vi "json editor worksheet.vi"() -> ()   [LabVIEW 2020]
uses:
  controls/step.ctl
  controls/step_type.ctl
  controls/write_read.ctl
panel:
  in  "exit without saving":bool
  in  "steps array out":T1[](array[typedef]) {"value" format="%.2f"}
  in  "exit and save":bool
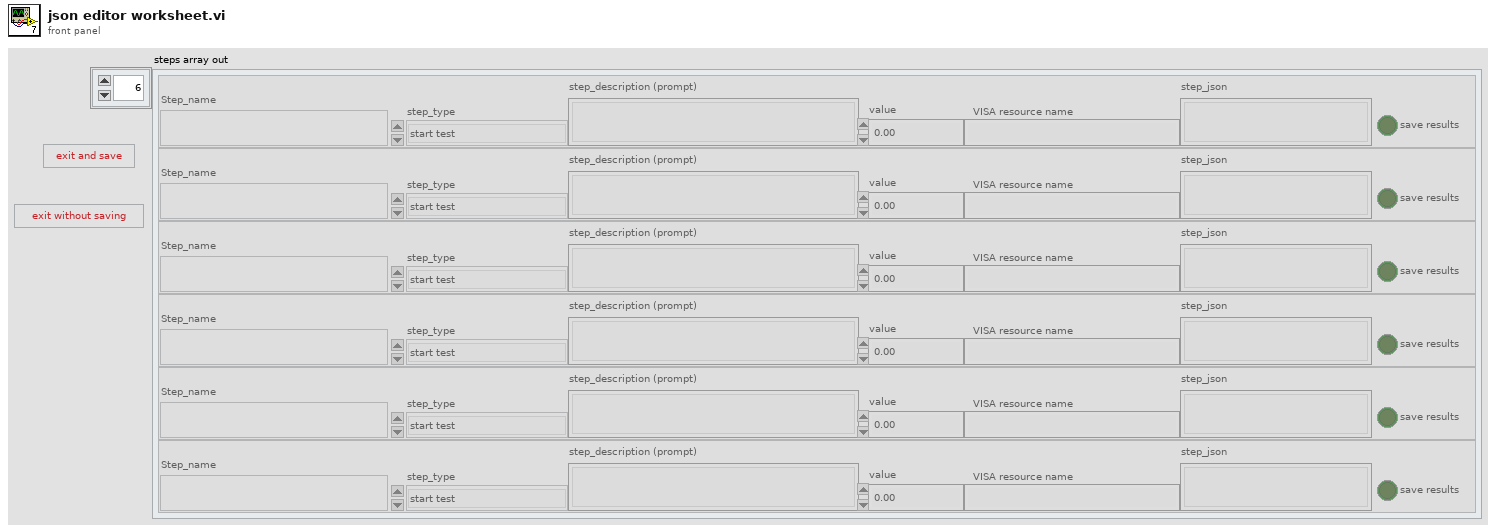
[diagram p1: front panel]
types:
  T1 = typedef "step.ctl" = cluster{"VISA resource name":string, "value":dbl, "step_description (prompt)":string, "step_json":string, "save results":bool, "step_type":T2, "Step_name":string}
  T2 = typedef "step_type.ctl" = enum16{"start test", "prompt", "sequence#", "12V power supply on_off", "set_hipot_V", "set_hipot_I_limit", "set_hipot_ramping (sec)", "read_hipot_V", "read_hipot_I", "set_daq", "read_daq", "flash uds", "wait", "record_pass_fail", "error_exit"}
  T3 = typedef "write_read.ctl" = enum16{"write", "read"}
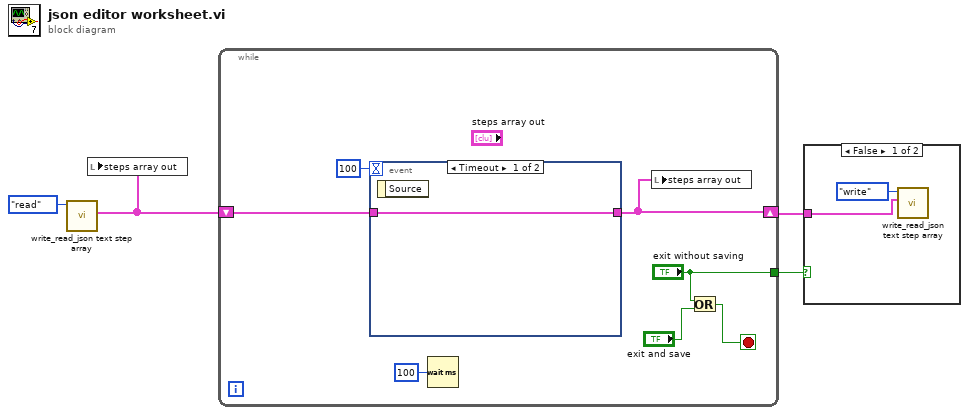
[diagram p0: block diagram]
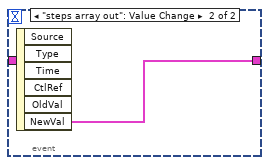
[diagram p3: hidden frame]
diagram:
  n1 = call "write_read_json text step array.vi"("write_read"=write_read."read") -> ("steps array out"=w3:T1[])  [unwired: 9 in, 1 out]
  n2 = local write "steps array out"(w3) -> ()
  n3 = while {
    shift-right: [w8] -> w2
    shift-left: w3 -> [w10]
    tunnel: ["exit without saving"] -> w1
    stop <- w6 stop-if-true
    n4 = event shown="[0] Timeout" {
      selector: _ -> [_ _]
      dyn-events: _ -> [_ _]
      timeout: 100 -> [_ _]
      tunnel: w10 -> [w12 _]
      tunnel: [w12 w13] -> w8
      event Timeout {
        n5 = event-data() -> ()  [unwired: 1 in, 1 out]
      }
      event "steps array out": Value Change {
        n6 = event-data() -> ("NewVal"=w13:T1[])  [unwired: 1 in, 5 out]
      }
    }
    n7 = Wait (ms)(milliseconds to wait=u32 100) -> ()  [unwired: 1 out]
    n8 = local write "steps array out"(w8) -> ()
    n9 = Or(x="exit without saving", y="exit and save") -> (x .or. y?=w6:bool)
  }
  n10 = case shown="False" w1 {
    tunnel: w2 -> [w14 _]
    frame False {
      n11 = call "write_read_json text step array.vi"("json_array_from_file"=w14, "write_read"=write_read."write") -> ()  [unwired: 8 in, 2 out]
    }
    frame True {
    }
  }
